vi "4 Way Switch.vi"() -> ()   [LabVIEW 2012]
uses:
  4 way slider.ctl
panel:
  out "Off":bool
  out "Standby":bool
  out "Hold":bool
  in  "Slide":T1 min=0 max=3 scale=0.0..3.0
  out "Run":bool
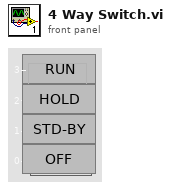
[diagram p1: front panel]
types:
  T1 = typedef "4 way slider.ctl" = i8
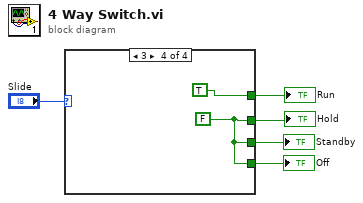
[diagram p0: block diagram]
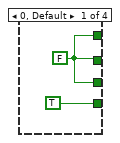
[diagram p2: hidden frame]
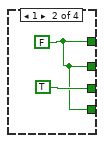
[diagram p3: hidden frame]
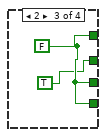
[diagram p4: hidden frame]
diagram:
  n1 = case shown="3" "Slide" {
    tunnel: [TRUE ("Run") w8 w11 w12] -> w4
    tunnel: [w6 w8 w11 TRUE ("Run")] -> w3
    tunnel: [w6 w8 TRUE ("Run") w12] -> w2
    tunnel: [w6 TRUE ("Run") w11 w12] -> w1
    frame 0, Default {
      w6 = FALSE ("Run")
    }
    frame 1 {
      w8 = FALSE ("Run")
    }
    frame 2 {
      w11 = FALSE ("Run")
    }
    frame 3 {
      w12 = FALSE ("Run")
    }
  }
  "Run" <- w3
  "Off" <- w4
  "Standby" <- w1
  "Hold" <- w2
